vi "Get Plugin Paths.vi"(8 "error in":errorcluster, 11 "measurement plugin service in":refnum<class "Fake Measurement Plugin.lvclass">) -> (0 "error out":errorcluster, 2 "plugin paths":T1, 3 "measurement plugin service out":refnum<class "Fake Measurement Plugin.lvclass">)   [LabVIEW 2020, in "MeasurementServerTests.lvlib" / "Measurement Plugin Service Tests.lvlib" / "Fake Measurement Plugin.lvclass"]
uses:
  Fake Measurement Plugin.lvclass
  Runtime/Measurements/Measurement Plugin Service/Plugin Paths.ctl
  Fake Measurement Plugin.lvclass/Fake Measurement Plugin.ctl
  Runtime/Measurements/Measurement Plugin Service/Measurement Plugin Service.lvclass
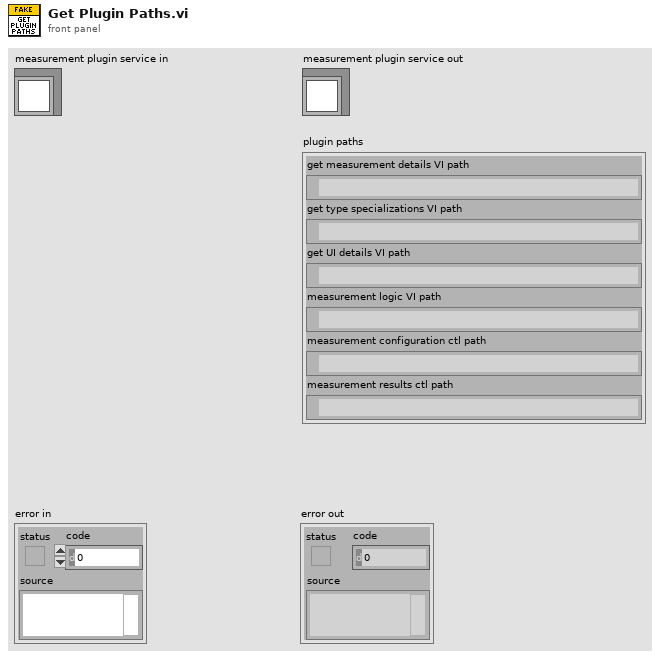
[diagram p1: front panel]
types:
  T1 = typedef "Plug-In SDK Measurement.lvlib/Measurement Plugin Service.lvclass/Plugin Paths.ctl" = cluster{"get measurement details VI path":path, "get type specializations VI path":path, "get UI details VI path":path, "measurement logic VI path":path, "measurement configuration ctl path":path, "measurement results ctl path":path}
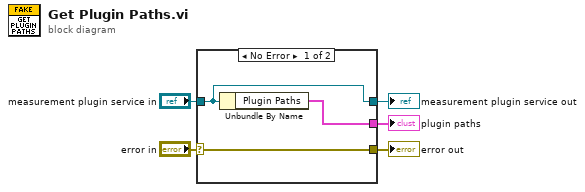
[diagram p0: block diagram]
diagram:
  n1 = case shown="No Error" "error in" {
    selector: "error in" -> [w8 w9]
    tunnel: [w8 w9] -> w4
    tunnel: "measurement plugin service in" -> [w6 w10]
    tunnel: [w7 _] -> w2
    tunnel: [w6 w10] -> w1
    frame No Error {
      n2 = Unbundle By Name(w6) -> ("Plugin Paths"=w7:T1)
    }
    frame Error {
    }
  }
  "error out" <- w4
  "measurement plugin service out" <- w1
  "plugin paths" <- w2
